vi "set_As_Liq.vi"(5 "ASLMFC1":dbl, 6 "Remote":bool=TRUE, 7 "Run":bool, 8 "Bubbler In":bool, 9 "Active":bool) -> ()   [LabVIEW 2011]
uses:
  low_level_proc/globals.vi
  editor_lib/Flow_Globals.vi
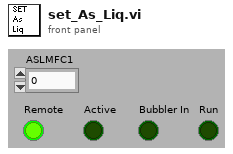
[diagram p1: front panel]
types:
  T1 = typedef "relaySpec.ctl" = cluster{"Card Index":u16, "Relay Index":u16}
  T2 = typedef "DA_Spec.ctl" = cluster{"Card Index":u16, "Channel Index":u16}
  T3 = typedef "AD_Spec.ctl" = u16
  T4 = cluster{"Relay Functions":cluster{"Remote":T1, "Active":T1, "Bubbler In":T1, "Run":T1}, "D/A Functions":cluster{"Flow":T2}, "Flow Ranges":cluster{"Flow (ASLMFC1)":u16}, "A/D Functions":cluster{"Flow":T3}}
  T5 = cluster{"Remote":T1, "Active":T1, "Bubbler In":T1, "Run":T1}
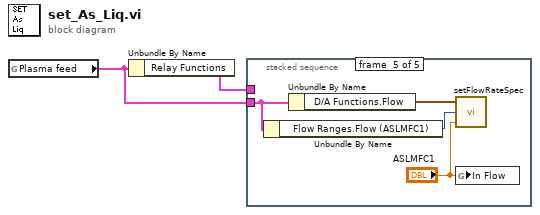
[diagram p0: block diagram]
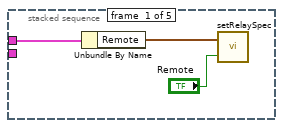
[diagram p2: hidden frame]
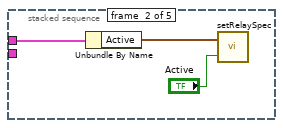
[diagram p3: hidden frame]
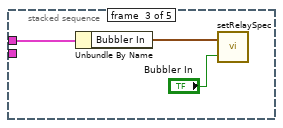
[diagram p4: hidden frame]
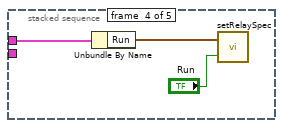
[diagram p5: hidden frame]
diagram:
  n1 = global read "globals.vi" "Plasma feed"() -> (w1:T4)
  n2 = Unbundle By Name(w1) -> ("Relay Functions"=w2:T5)
  n3 = stacked-sequence {
    tunnel: w2 -> [w3 w6 w9 w12 _]
    tunnel: w1 -> [_ _ _ _ w15]
    frame #0 {
      n4 = Unbundle By Name(w3) -> ("Remote"=w4:T1)
      n5 = call "setRelaySpec.vi"("Relay Status"="Remote", "RelaySpec"=w4) -> ()  [unwired: 1 in]
    }
    frame #1 {
      n6 = Unbundle By Name(w6) -> ("Active"=w7:T1)
      n7 = call "setRelaySpec.vi"("Relay Status"="Active", "RelaySpec"=w7) -> ()  [unwired: 1 in]
    }
    frame #2 {
      n8 = Unbundle By Name(w9) -> ("Bubbler In"=w10:T1)
      n9 = call "setRelaySpec.vi"("Relay Status"="Bubbler In", "RelaySpec"=w10) -> ()  [unwired: 1 in]
    }
    frame #3 {
      n10 = Unbundle By Name(w12) -> ("Run"=w13:T1)
      n11 = call "setRelaySpec.vi"("Relay Status"="Run", "RelaySpec"=w13) -> ()  [unwired: 1 in]
    }
    frame #4 {
      n12 = Unbundle By Name(w15) -> ("Flow Ranges.Flow (ASLMFC1)"=w17:u16)
      n13 = Unbundle By Name(w15) -> ("D/A Functions.Flow"=w16:T2)
      n14 = call "setFlowRateSpec.vi"("Flow Rate (sccm)"="ASLMFC1", "Flow range Index"=w17, "D/A Card"=w16) -> ()  [unwired: 2 in]
      n15 = global write "Flow_Globals.vi" "In Flow"("ASLMFC1") -> ()
    }
  }
